vi "MGCC_StaEst_Add_noise.vi"(0 "spn":dbl=1.0 format="%0.2f", 1 "sqn":dbl=1.0 format="%0.2f", 2 "svn":dbl=1.0 format="%0.2f", 3 "Node":i32) -> (5 "sspn":dbl[][](array[numeric]), 6 "ssvn":dbl[][](array[numeric]), 7 "ssqn":dbl[][](array[numeric]))   [LabVIEW 2016]
uses:
  <vilib>/ptbypt/NI_PtbyPt.lvlib
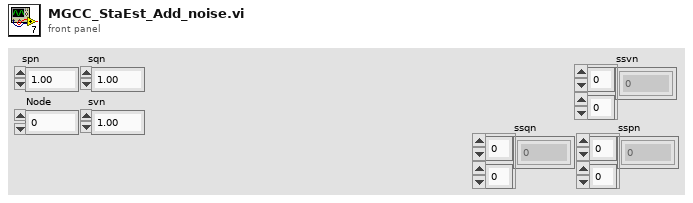
[diagram p1: front panel]
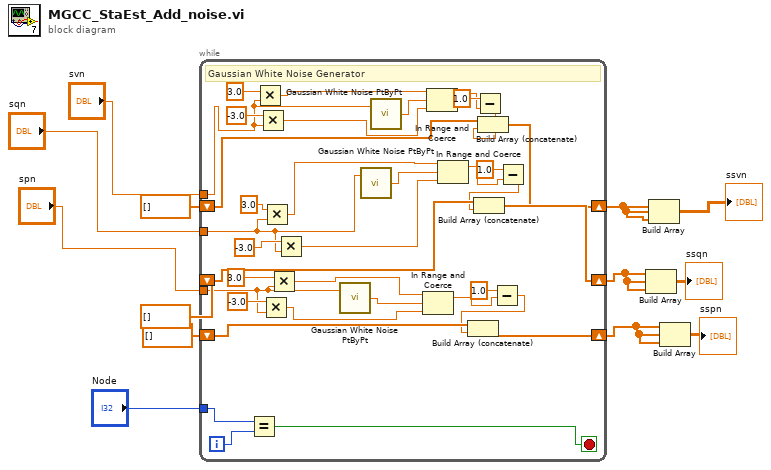
[diagram p0: block diagram]
diagram:
  n1 = while {
    tunnel: "spn" -> [w27]
    shift-right: [w44] -> w3
    shift-left: dbl[] [] -> [w49]
    tunnel: "Node" -> [w48]
    tunnel: "svn" -> [w35]
    tunnel: "sqn" -> [w28]
    shift-right: [w43] -> w4
    shift-left: dbl[] [] -> [w45]
    shift-right: [w42] -> w6
    shift-left: dbl[] [] -> [w41]
    i -> [w47]
    stop <- w46 stop-if-true
    # "Gaussian White Noise Generator"
    n2 = Equal?(x=w48, y=w47) -> (x = y?=w46:bool)
    n3 = Multiply(x=3.0, y=w35) -> (x*y=w34:dbl)
    n4 = Multiply(x=-3.0, y=w35) -> (x*y=w33:dbl)
    n5 = Multiply(x=-3.0, y=w27) -> (x*y=w23:dbl)
    n6 = Multiply(x=3.0, y=w28) -> (x*y=w26:dbl)
    n7 = Multiply(x=3.0, y=w27) -> (x*y=w24:dbl)
    n8 = Multiply(x=-3.0, y=w28) -> (x*y=w25:dbl)
    n9 = call <vilib>:"Gaussian White Noise PtByPt.vi"("standard deviation"=w27) -> ("Gaussian white noise"=w40:dbl)  [unwired: 2 in]
    n10 = call <vilib>:"Gaussian White Noise PtByPt.vi"("standard deviation"=w28) -> ("Gaussian white noise"=w39:dbl)  [unwired: 2 in]
    n11 = call <vilib>:"Gaussian White Noise PtByPt.vi"("standard deviation"=w35) -> ("Gaussian white noise"=w38:dbl)  [unwired: 2 in]
    n12 = In Range and Coerce(upper limit=w24, x=w40, lower limit=w23) -> (coerced(x)=w19:dbl)  [unwired: 1 out]
    n13 = In Range and Coerce(upper limit=w34, x=w38, lower limit=w33) -> (coerced(x)=w15:dbl)  [unwired: 1 out]
    n14 = In Range and Coerce(upper limit=w26, x=w39, lower limit=w25) -> (coerced(x)=w17:dbl)  [unwired: 1 out]
    n15 = Subtract(x=1.0, y=w15) -> (x-y=w14:dbl)
    n16 = Build Array (concatenate)(w41, w14) -> (w42:dbl[])
    n17 = Subtract(x=1.0, y=w19) -> (x-y=w18:dbl)
    n18 = Build Array (concatenate)(w49, w18) -> (w44:dbl[])
    n19 = Subtract(x=1.0, y=w17) -> (x-y=w16:dbl)
    n20 = Build Array (concatenate)(w45, w16) -> (w43:dbl[])
  }
  n21 = Build Array(w4, w4, w4) -> (→"ssqn":dbl[][])
  n22 = Build Array(w6, w6, w6) -> (→"ssvn":dbl[][])
  n23 = Build Array(w3, w3, w3) -> (→"sspn":dbl[][])
